vi "WF3.vi"(6 "TxWaveformStyle":i32, 8 "TxFreqIndex":i32, 9 "BeamStyleIndex":i32, 10 "Timeout (ms)":i32=40000000, 11 "connection ID in":refnum<k5>) -> (2 "Timeout (ms) out":i32, 3 "connection ID out":refnum<k5>)   [LabVIEW 2016]
uses:
  TemperatureMeasure/Thermal_type.vi
panel:
  out "TxFreqIndex":dbl[](array[numeric])
  out "NumTxFreq":dbl
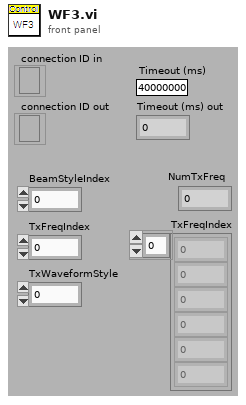
[diagram p1: front panel]
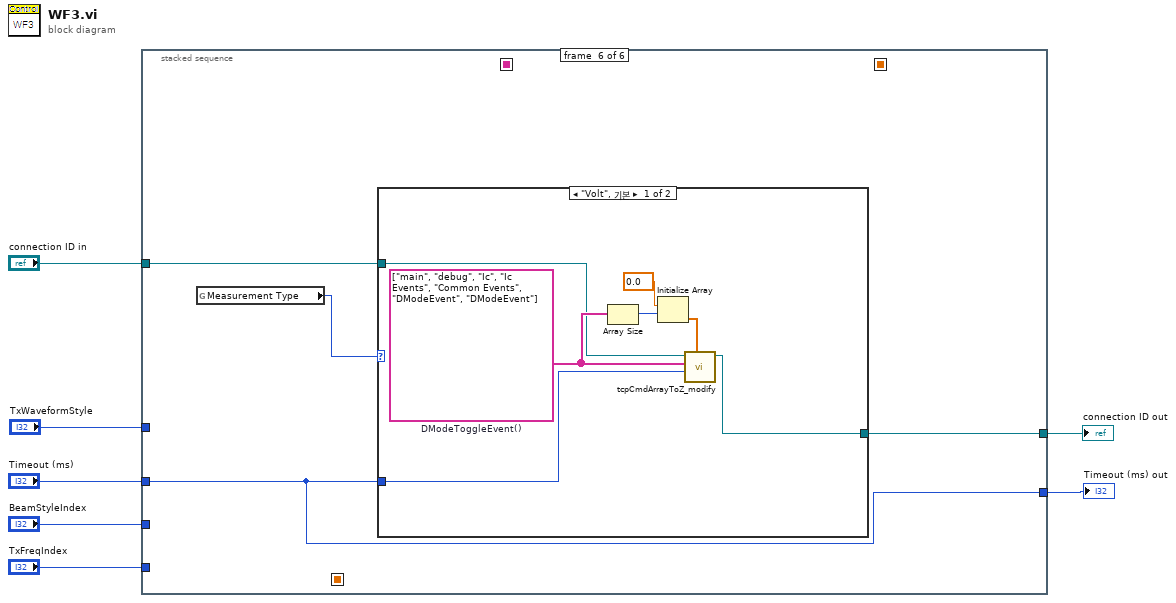
[diagram p0: block diagram]
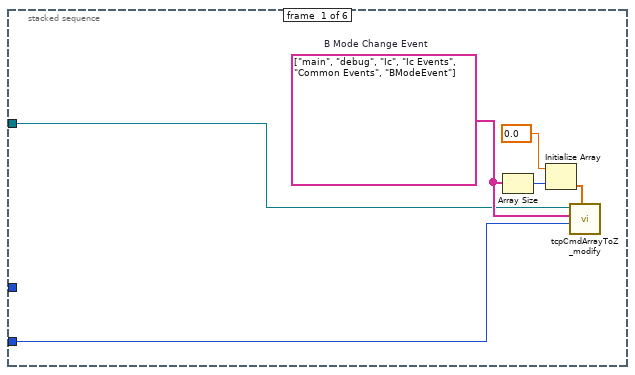
[diagram p2: hidden frame]
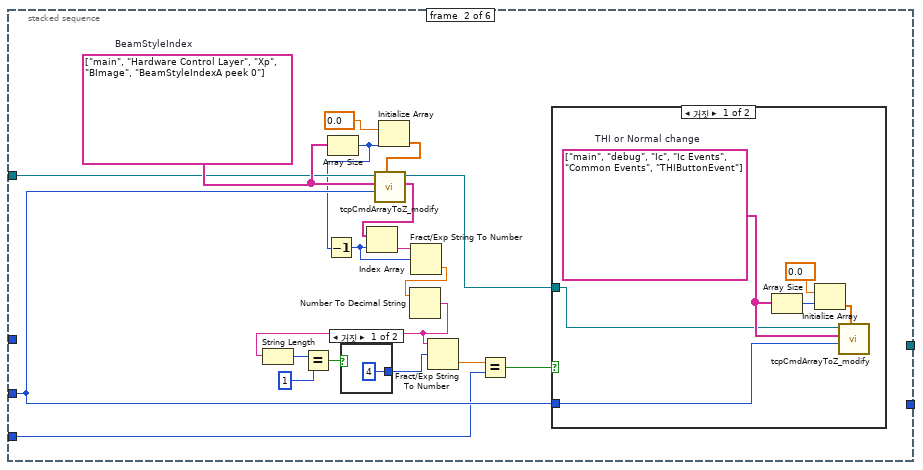
[diagram p3: hidden frame]
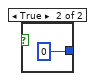
[diagram p4: hidden frame]
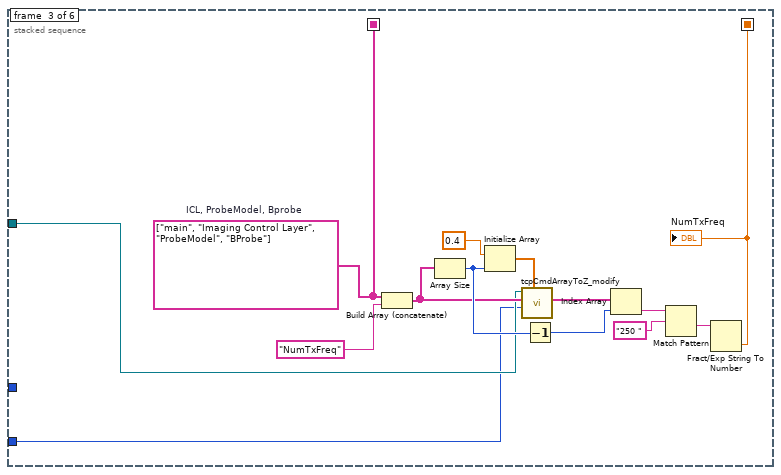
[diagram p6: hidden frame]
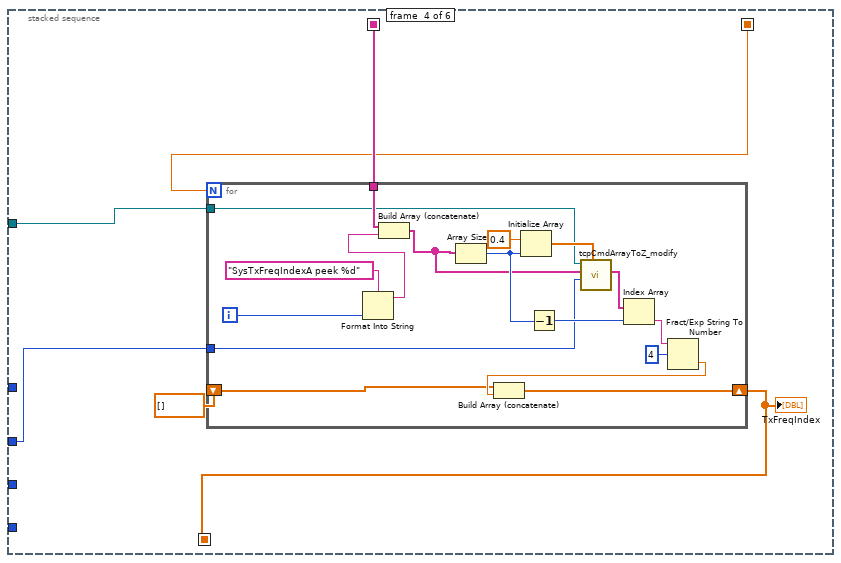
[diagram p7: hidden frame]
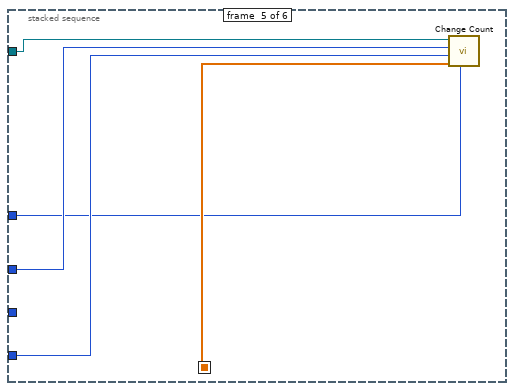
[diagram p8: hidden frame]
diagram:
  n1 = stacked-sequence {
    seq-local: [_ _ w44 _ _ _] -> [_ _ _ w59 _ _]
    seq-local: [_ _ w43 _ _ _] -> [_ _ _ w58 _ _]
    seq-local: [_ _ _ w57 _ _] -> [_ _ _ _ w80 _]
    tunnel: "connection ID in" -> [w9 w24 w42 w56 w82 w84]
    tunnel: "Timeout (ms)" -> [w8 w32 w41 w55 w79 w85]
    tunnel: [_ _ _ _ _ w86] -> w5
    tunnel: [_ _ _ _ _ w85] -> w4
    tunnel: "BeamStyleIndex" -> [_ w25 _ _ _ _]
    tunnel: "TxFreqIndex" -> [_ _ _ _ w81 _]
    tunnel: "TxWaveformStyle" -> [_ _ _ _ w78 _]
    frame #0 {
      w13 = string[] ["main", "debug", "Ic", "Ic Events", "Common Events", "BModeEvent"]  # B Mode Change Event
      n2 = Array Size(array=w13) -> (size(s)=w10:i32)
      n3 = Initialize Array(sgl 0.0 ("element"), w10) -> (w12:sgl[])
      n4 = call "tcpCmdArrayToZ_modify.vi"("Delay (sec)"=w12, "Timeout (ms)"=w8, "Command array"=w13, "connection ID in"=w9) -> ()  [unwired: 3 in, 5 out]
    }
    frame #1 {
      w31 = string[] ["main", "Hardware Control Layer", "Xp", "BImage", "BeamStyleIndexA peek 0"]  # BeamStyleIndex
      n5 = Array Size(array=w31) -> (size(s)=w17:i32)
      n6 = Decrement(x=w17) -> (x-1=w16:i32)
      n7 = Initialize Array(sgl 0.0 ("element"), w17) -> (w29:sgl[])
      n8 = call "tcpCmdArrayToZ_modify.vi"("Delay (sec)"=w29, "Timeout (ms)"=w32, "Command array"=w31, "connection ID in"=w24) -> ("Receive array"=w18:string[], "connection ID out"=w27:refnum<k5>)  [unwired: 3 in, 3 out]
      n9 = Index Array(array=w18, index=w16) -> (element=w19:string)
      n10 = Fract/Exp String To Number(string=w19, offset=w16) -> (number=w15:dbl)  [unwired: 2 in, 1 out]
      n11 = Number To Decimal String(number=w15) -> (decimal integer string=w14:string)  [unwired: 1 in]
      n12 = String Length(string=w14) -> (length=w23:i32)
      n13 = Equal?(x=w23, y=1) -> (x = y?=w21:bool)
      n14 = case shown="거짓" w21 {
        tunnel: [4 0] -> w20
        frame False {
        }
        frame True {
        }
      }
      n15 = Fract/Exp String To Number(string=w14, offset=w20) -> (number=w28:dbl)  [unwired: 2 in, 1 out]
      n16 = Equal?(x=w28, y=w25) -> (x = y?=w26:bool)
      n17 = case shown="거짓" w26 {
        tunnel: w27 -> [w36 _]
        tunnel: w32 -> [w35 _]
        frame False {
          w37 = string[] ["main", "debug", "Ic", "Ic Events", "Common Events", "THIButtonEvent"]  # THI or Normal change
          n18 = Array Size(array=w37) -> (size(s)=w40:i32)
          n19 = Initialize Array(sgl 0.0 ("element"), w40) -> (w38:sgl[])
          n20 = call "tcpCmdArrayToZ_modify.vi"("Delay (sec)"=w38, "Timeout (ms)"=w35, "Command array"=w37, "connection ID in"=w36) -> ()  [unwired: 3 in, 5 out]
        }
        frame True {
        }
      }
    }
    frame #2 {
      w44 = string[] ["main", "Imaging Control Layer", "ProbeModel", "BProbe"]  # ICL, ProbeModel, Bprobe
      n21 = Build Array (concatenate)(w44, "NumTxFreq") -> (w45:string[])
      n22 = Array Size(array=w45) -> (size(s)=w47:i32)
      n23 = Initialize Array(0.4 ("원소"), w47) -> (w53:dbl[])
      n24 = call "tcpCmdArrayToZ_modify.vi"("Delay (sec)"=w53, "Timeout (ms)"=w41, "Command array"=w45, "connection ID in"=w42) -> ("Receive array"=w48:string[])  [unwired: 3 in, 4 out]
      n25 = Decrement(x=w47) -> (x-1=w51:i32)
      n26 = Index Array(array=w48, index=w51) -> (element=w52:string)
      n27 = Match Pattern(string=w52, regular expression="250 " ("정규식")) -> (after substring=w50:string)  [unwired: 1 in, 3 out]
      n28 = Fract/Exp String To Number(string=w50) -> (number=w43:dbl)  [unwired: 3 in, 1 out]
      "NumTxFreq" <- w43
    }
    frame #3 {
      n29 = for {
        N: w58 -> [_]
        tunnel: w59 -> [w66]
        shift-right: [w64] -> w57
        shift-left: dbl[] [] -> [w63]
        tunnel: w56 -> [w62]
        tunnel: w55 -> [w61]
        i -> [w77]
        n30 = Format Into String(format string="SysTxFreqIndexA peek %d" ("초기 문자열"), w77) -> (resulting string=w67:string)  [unwired: 2 in, 1 out]
        n31 = Build Array (concatenate)(w66, w67) -> (w65:string[])
        n32 = Array Size(array=w65) -> (size(s)=w73:i32)
        n33 = Initialize Array(0.4 ("원소"), w73) -> (w71:dbl[])
        n34 = Decrement(x=w73) -> (x-1=w72:i32)
        n35 = call "tcpCmdArrayToZ_modify.vi"("Delay (sec)"=w71, "Timeout (ms)"=w61, "Command array"=w65, "connection ID in"=w62) -> ("Receive array"=w74:string[])  [unwired: 3 in, 4 out]
        n36 = Index Array(array=w74, index=w72) -> (element=w70:string)
        n37 = Fract/Exp String To Number(string=w70, offset=4 ("오프셋")) -> (number=w68:dbl)  [unwired: 2 in, 1 out]
        n38 = Build Array (concatenate)(w63, w68) -> (w64:dbl[])
      }
      "TxFreqIndex" <- w57
    }
    frame #4 {
      n39 = call "Change Count.vi"("connection ID in"=w82, "Timeout (ms)"=w79, 3:"TxFreqIndex"=w81, "TxWaveformStyle"=w78, 5:"TxFreqIndex"=w80) -> ()  [unwired: 3 in, 1 out]
    }
    frame #5 {
      n40 = global read "Thermal_type.vi" "Measurement Type"() -> (w83:enum32{"Volt", "SA"})
      n41 = case shown="\"Volt\", 기본" w83 {
        tunnel: [w89 w94] -> w86
        tunnel: w85 -> [w88 _]
        tunnel: w84 -> [w87 w94]
        frame "Volt", Default {
          w90 = string[] ["main", "debug", "Ic", "Ic Events", "Common Events", "DModeEvent", "DModeEvent"]  # DModeToggleEvent()
          n42 = Array Size(array=w90) -> (size(s)=w93:i32)
          n43 = Initialize Array(sgl 0.0 ("element"), w93) -> (w91:sgl[])
          n44 = call "tcpCmdArrayToZ_modify.vi"("Delay (sec)"=w91, "Timeout (ms)"=w88, "Command array"=w90, "connection ID in"=w87) -> ("connection ID out"=w89:refnum<k5>)  [unwired: 3 in, 4 out]
        }
        frame "SA" {
        }
      }
    }
  }
  "connection ID out" <- w5
  "Timeout (ms) out" <- w4
